vi "MCSHostTest.vi"() -> ()   [LabVIEW 2014]
uses:
  <vilib>/FPGAPlugInAG/PXI-7852R/niLvFpga_Open_PXI-7852R.vi
  <vilib>/rvi/interface/common/dynamic/niFpgaDynamicAddResources.vi
  <vilib>/rvi/interface/common/niFpgaWaitOnOcc.vi
  <vilib>/Utility/error.llb/Error Cluster From Error Code.vi
  <vilib>/rvi/errors/niLvFpgaAdjustHostInterfaceError.vi
  <vilib>/FPGAPlugInAG/Dynamic/niLvFpga_Close_Dynamic.vi
  <vilib>/rvi/interface/nirviOpenFPGA/nirviOpenFPGA.xnode
  FPGA Bitfiles/TiTaProj_DAF_103.lvbitx
  <vilib>/rvi/interface/nirviMethod/nirviMethod.xnode
  <vilib>/rvi/interface/nirviReadWriteControl/nirviReadWriteControl.xnode
  <vilib>/rvi/interface/nirviCloseFPGA/nirviCloseFPGA.xnode
  NiFpgaLv.dll
  <vilib>/rvi/interface/Simulation/niFpgaSimulationCallBeginRW.vi
  <vilib>/rvi/errors/niLvFpgaMergeErrorWithErrorCode.vi
  <vilib>/FPGAPlugInAG/Dynamic/niLvFpga_ReadFifo_Dynamic.vi
  <vilib>/FPGAPlugInAG/Dynamic/niLvFpga_ConfigureFifo_Dynamic.vi
panel:
  out "TRSArray":u32[][][](array[numeric])
  in  "SendHaltAbort":bool
  out "TRSdataUntouchedOut":u32[](array[numeric]) format="%032b"
  out "VoltArray":u32[](array[numeric]) format="%032b"
  in  "AnalyseData":bool
  out "ReadData":u32[](array[numeric]) format="%032b"
  out "SavedData":u32[](array[numeric]) format="%032b"
  in  "SendCommand":bool
  out "MCSQuWriteTimeout":bool
  out "DACQuWriteTimeout":bool
  out "MCSerrorcount":i8
  in  "cmdByHost":T1(ring)
  out "MCSstate":enum16{"idle", "scanning", "done", "error"}(ring)
  out "seqState":T1(ring)
  in  "nOfBunches":i32
  in  "nOfBins":u32=4000
  in  "delay(ticks)":u32=1000
  in  "MCSSelectTrigger":T2(ring)=enum."Int0"
  in  "hostConfirmsHzOffsetIsSet":bool
  in  "halt":bool
  in  "abort":bool
  in  "measVoltTimeout(10ns)":i32
  in  "measVoltPulseLength(25ns)":i32
  in  "waitAfterReset(25nsTicks)":u16
  in  "waitForKepco(25nsTicks)":u16
  in  "heinzingerControl":T3(ring)
  in  "invertScan":bool
  in  "nOfScans":i32=6
  in  "nOfSteps":i32=6
  in  "start":i32 format="%024b"
  in  "stepSize":i32=2048 format="%024b"
  in  "VoltOrScaler?":bool
  out "measVoltState":T4(ring)
  in  "SetParameters":bool
  in  "stop":bool
  # "cmd is send when control in ui changes"
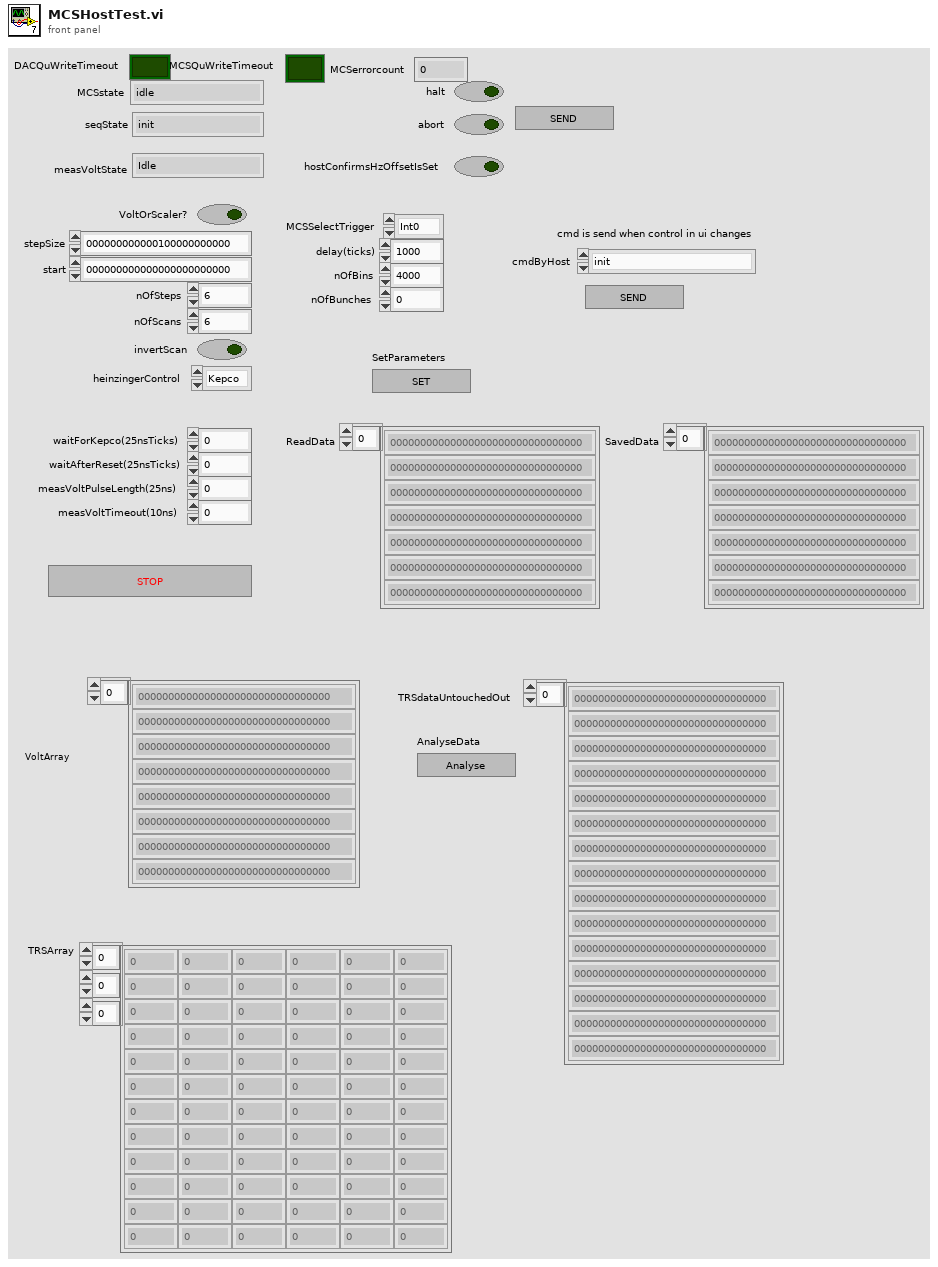
[diagram p1: front panel]
types:
  T1 = enum16{"init", "idle", "measureOffset", "measureTrack", "measComplete", "error"}
  T2 = enum8{"Ext0", "Ext1", "Ext2", "Ext3", "Ext4", "Ext5", "Ext6", "Ext7", "Int0", "Int1", "Int2", "Int3", "Int4", "Int5", "Int6", "Int7"}
  T3 = enum8{"Kepco", "Heinzinger0", "Heinzinger1", "Heinzinger2"}
  T4 = enum16{"Idle", "sendMeasRequest", "waitUntilDone", "done"}
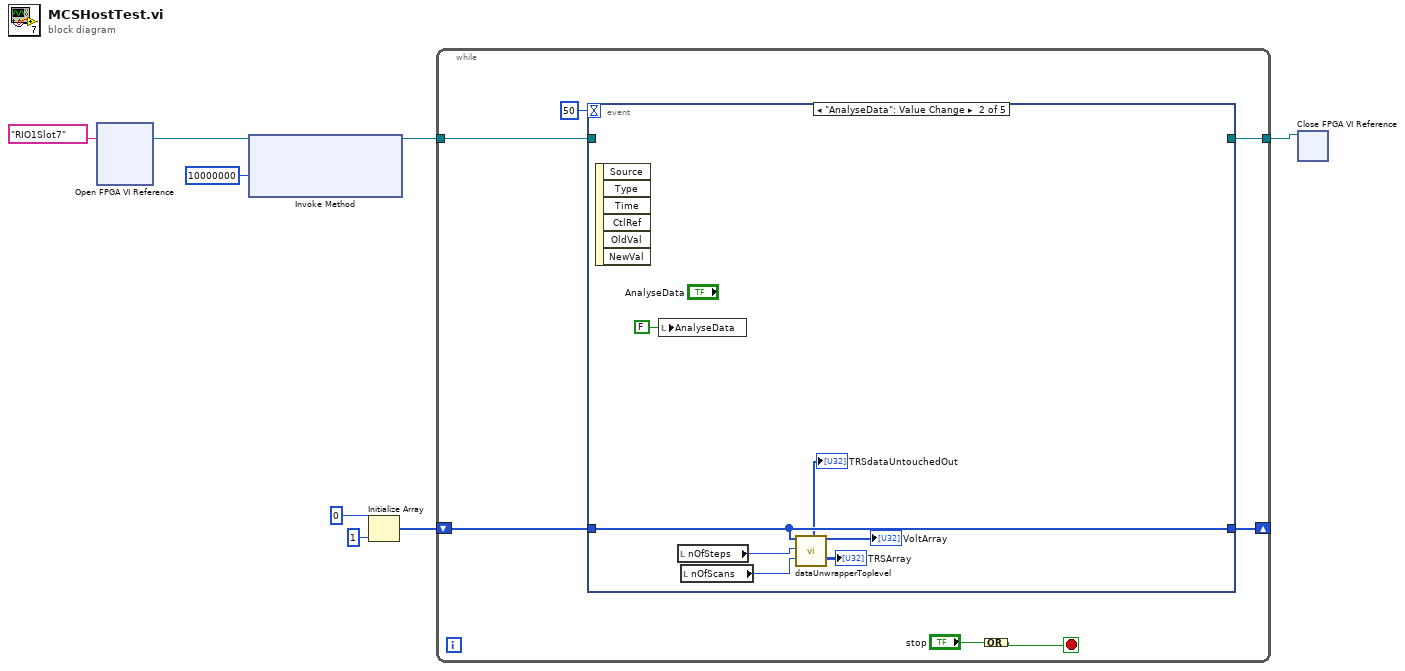
[diagram p0: block diagram]
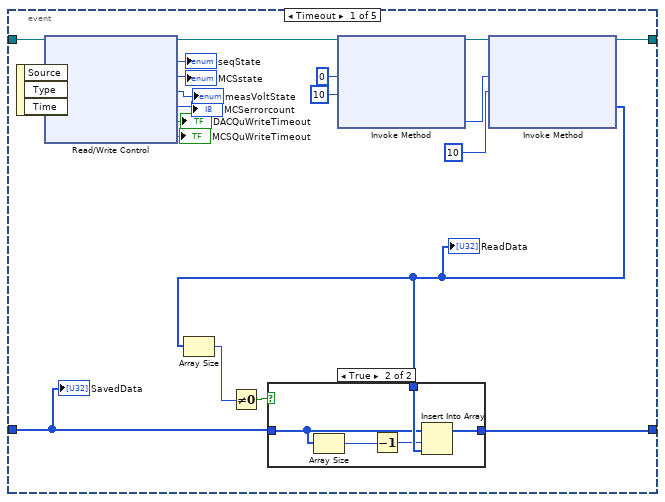
[diagram p2: hidden frame]
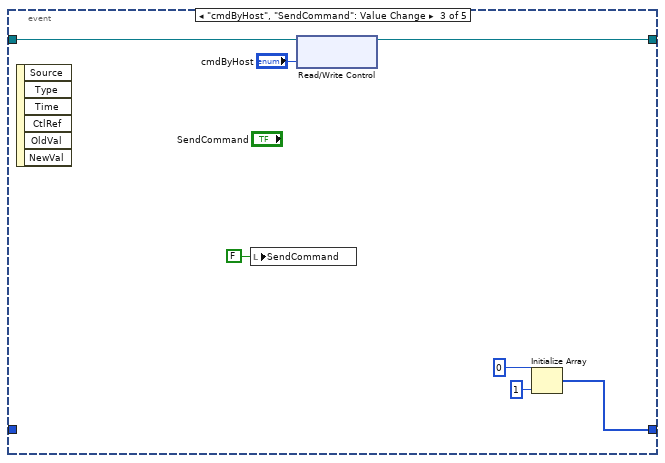
[diagram p4: hidden frame]
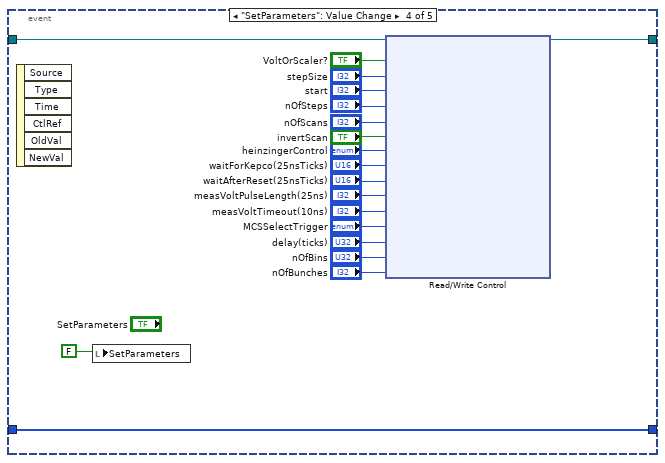
[diagram p5: hidden frame]
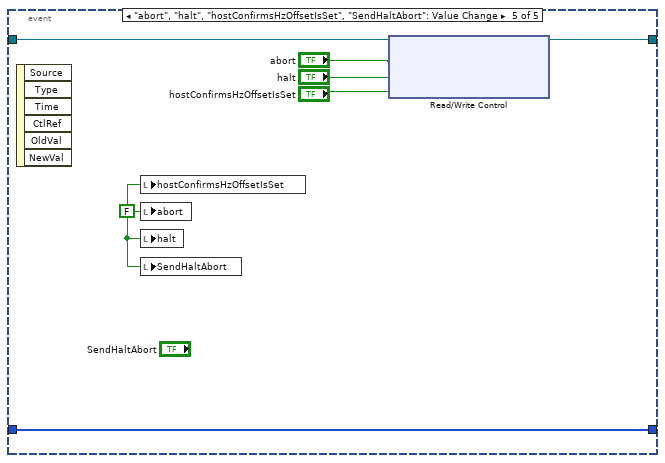
[diagram p6: hidden frame]
diagram:
  n1 = xnode "Open FPGA VI Reference"("resource name"=tag "RIO1Slot7") -> ("FPGA VI Reference Out"=w8:refnum<k20>)  [unwired: 1 in, 1 out]
  n2 = xnode "Invoke Method"("FPGA VI Reference In"=w8, "Requested Depth"=u32 10000000) -> ("FPGA VI Reference Out"=w5:refnum<k20>)  [unwired: 1 in, 2 out]
  n3 = Initialize Array(u32 0 ("element"), 1 ("dimension size")) -> (w1:u32[])
  n4 = while {
    tunnel: w5 -> [w12]
    tunnel: [w11] -> w7
    shift-right: [w10] -> _
    shift-left: w1 -> [w9]
    stop <- w13 stop-if-true
    n5 = event shown="[1] \"AnalyseData\": Value Change" {
      selector: _ -> [_ _ _ _ _]
      dyn-events: _ -> [_ _ _ _ _]
      timeout: 50 -> [_ _ _ _ _]
      tunnel: w12 -> [w34 _ w54 w72 w80]
      tunnel: [w28 _ w53 w56 w79] -> w11
      tunnel: [w18 w46 w48 w55 w75] -> w10
      tunnel: w9 -> [w17 w46 _ w55 w75]
      event Timeout {
        n6 = event-data() -> ()  [unwired: 1 in, 3 out]
        n7 = xnode "Read/Write Control"("FPGA VI Reference In"=w34) -> ("FPGA VI Reference Out"=w32:refnum<k20>, "seqState"=→"seqState":T1, "MCSstate"=→"MCSstate":enum16{"idle", "scanning", "done", "error"}, "measVoltState"=→"measVoltState":T4, "MCSerrorcount"=→"MCSerrorcount":i8, "DACQuWriteTimeout"=→"DACQuWriteTimeout":bool, "MCSQuWriteTimeout"=→"MCSQuWriteTimeout":bool)  [unwired: 1 in, 1 out]
        n8 = xnode "Invoke Method"("FPGA VI Reference In"=w32, "Number of Elements"=u32 0, "Timeout (ms)"=10) -> ("FPGA VI Reference Out"=w31:refnum<k20>, "Elements Remaining"=w27:u32)  [unwired: 1 in, 2 out]
        n9 = xnode "Invoke Method"("FPGA VI Reference In"=w31, "Number of Elements"=w27, "Timeout (ms)"=10) -> ("FPGA VI Reference Out"=w28:refnum<k20>, "Data"=w16:u32[])  [unwired: 1 in, 2 out]
        "ReadData" <- w16
        n10 = Array Size(array=w16) -> (size(s)=w19:i32)
        n11 = Not Equal To 0?(x=w19) -> (x != 0?=w20:bool)
        n12 = case shown="True" w20 {
          tunnel: w16 -> [_ w40]
          tunnel: [w35 w39] -> w18
          tunnel: w17 -> [w35 w38]
          frame False {
          }
          frame True {
            n13 = Array Size(array=w38) -> (size(s)=w37:i32)
            n14 = Decrement(x=w37) -> (x-1=w36:i32)
            n15 = Insert Into Array(array=w38, index=w36, new element=w40) -> (w39:u32[])
          }
        }
        "SavedData" <- w17
      }
      event "AnalyseData": Value Change {
        n16 = event-data() -> ()  [unwired: 1 in, 6 out]
        n17 = local write "AnalyseData"(FALSE ("AnalyseData")) -> ()
        n18 = local read "nOfSteps"() -> (w45:i32)
        n19 = local read "nOfScans"() -> (w44:i32)
        n20 = call "dataUnwrapperToplevel.vi"("dataIn"=w46, "nOfSteps"=w45, "nOfScans"=w44) -> ("DataUntouchedOut"=→"TRSdataUntouchedOut":u32[], "VoltArray"=→"VoltArray":u32[], "TRSArray"=→"TRSArray":u32[][][])  [unwired: 13 in, 1 out]
      }
      event "cmdByHost", "SendCommand": Value Change {
        n21 = event-data() -> ()  [unwired: 1 in, 6 out]
        n22 = local write "SendCommand"(FALSE ("SendCommand")) -> ()
        n23 = xnode "Read/Write Control"("FPGA VI Reference In"=w54, "cmdByHost"="cmdByHost") -> ("FPGA VI Reference Out"=w53:refnum<k20>)  [unwired: 1 in, 1 out]
        n24 = Initialize Array(u32 0 ("element"), 1 ("dimension size")) -> (w48:u32[])
      }
      event "SetParameters": Value Change {
        n25 = event-data() -> ()  [unwired: 1 in, 6 out]
        n26 = local write "SetParameters"(FALSE ("SetParameters")) -> ()
        n27 = xnode "Read/Write Control"("FPGA VI Reference In"=w72, "VoltOrScaler?"="VoltOrScaler?", "stepSize"="stepSize", "start"="start", "nOfSteps"="nOfSteps", "nOfScans"="nOfScans", "invertScan"="invertScan", "heinzingerControl"="heinzingerControl", "waitForKepco(25nsTicks)"="waitForKepco(25nsTicks)", "waitAfterReset(25nsTicks)"="waitAfterReset(25nsTicks)", "measVoltPulseLength(25ns)"="measVoltPulseLength(25ns)", "measVoltTimeout(10ns)"="measVoltTimeout(10ns)", "MCSSelectTrigger"="MCSSelectTrigger", "delay(ticks)"="delay(ticks)", "nOfBins"="nOfBins", "nOfBunches"="nOfBunches") -> ("FPGA VI Reference Out"=w56:refnum<k20>)  [unwired: 1 in, 1 out]
      }
      event "abort", "halt", "hostConfirmsHzOffsetIsSet", "SendHaltAbort": Value Change {
        w74 = FALSE ("abort")
        n28 = event-data() -> ()  [unwired: 1 in, 6 out]
        n29 = local write "hostConfirmsHzOffsetIsSet"(w74) -> ()
        n30 = local write "abort"(w74) -> ()
        n31 = local write "halt"(w74) -> ()
        n32 = local write "SendHaltAbort"(w74) -> ()
        n33 = xnode "Read/Write Control"("FPGA VI Reference In"=w80, "abort"="abort", "halt"="halt", "hostConfirmsHzOffsetIsSet"="hostConfirmsHzOffsetIsSet") -> ("FPGA VI Reference Out"=w79:refnum<k20>)  [unwired: 1 in, 1 out]
      }
    }
    n34 = Compound Arithmetic op=OR("stop") -> (w13:bool)
  }
  n35 = xnode "Close FPGA VI Reference"("FPGA VI Reference In"=w7) -> ()  [unwired: 1 in, 1 out]
